vi "MultiChannelType_2D-Array-SGL.vi"(9 "error in":errorcluster, 11 "Array in":sgl[][](array[numeric])) -> (1 "error out":errorcluster, 2 "MultiChannelType":csg, 3 "Array out":sgl[][](array[numeric]))   [LabVIEW 2020, in "OpenLvVision_OpenCv.lvlib"]
uses:
  OpenLvVision_OpenCv.lvlib
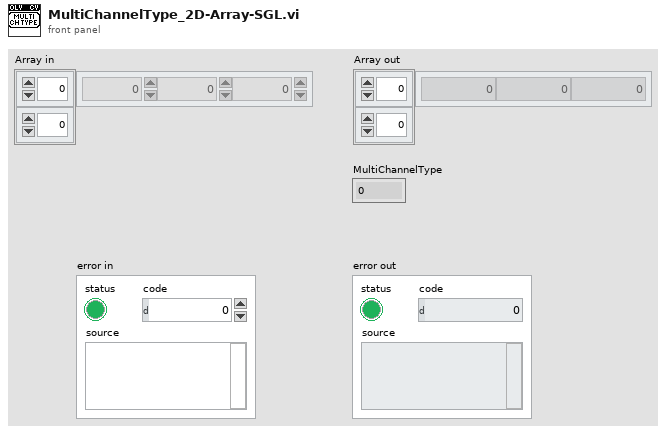
[diagram p1: front panel]
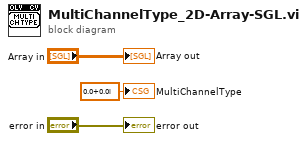
[diagram p0: block diagram]
diagram:
  "error out" <- "error in"
  "Array out" <- "Array in"
  "MultiChannelType" <- csg 0.0+0.0i
